vi "Breakdown Acoustics Controls.vi"() -> ()   [LabVIEW 2013]
doc: "Recommended Input Signal: 10 Hz, 1.8 Vpp, sine wave\n\nThis example requires NI-Scope 3.3 or later.\nDevices Supported: NI 5112, NI 5620, NI 5621, NI 5122, NI 5124, NI 5922, NI 5114, NI 5142\n\nVI Description:\n\nThis example demonstrates using continuous acquisition to fetch a user-defined, but quite large record of data all while continuously streaming the data to a binary file using the Win32 File I/O VIs. The digitizer is configured using the Configure Vertical and Configure Horizontal VI's. Auto setup in this case may not be useful, as it may choose a horizontal rate that exceeds the computer's streaming capabilities.\n\nIn this example, continuous acquisition is used. This allows the user to start the digitizer, and continuously fetch data without losing any points. This is accomplished by configuring a software trigger and never sending the software trigger. Therefore, the digitizer will continuously acquire data into its onboard memory until Abort or Close is called.\n\nThe producer loop continuously fetches data from onboard memory into the LabVIEW memory using DMA transfers. This data is placed into a queue in order to efficiently transfer the data to a parallel consumer loop where it is written file. If the sampling rate is low, the computer can fetch all the data from the digitizer, so data is never overwritten. However, at faster sampling rates, the computer will not be able to fetch the data before it is overwritten by new data. This results in the \"data overwritten\" error.\n\nThe consumer loop continuously empties data from the queue and writes data to disk using the Win32 Write File.vi. The file is opened using the Win32 Open File.vi, which disables Windows caching during the write process, resulting in increased performance. However when Windows caching is disabled, <b>data must be written to file in a multiple of the sector size of the disk (typically 512 bytes).</b>"
uses:
  <vilib>/Utility/error.llb/DialogType.ctl
  Breakdown Acoustics Controls/UDP Heartbeat Globals.vi
  <vilib>/Waveform/WDTFileIO.llb/ Write Waveforms to File (1D).vi
  Breakdown Acoustics Controls.lvlib
panel:
  out "Spark!":bool
  out "Spark Flag Updater\nHeartbeat":bool
  out "# DAQ Restarts":i32
  out "# Triggers":i32
  in  "Force Trigger":bool
  out "Triggered":bool
  in  "Tab Control":T1(tab)
  in  "Max Queue Size":i32=8
  in  "Samples Per Channel":i32=5120 caption="Max Points Per Fetch" step=1048576
  in  "Configuration File":path=path "\\\\beams-utility\\mta_archive$/mtarflv_shared/Microphone DAQ/LabVIEW/VI/Shared/SCM_without_Cu_windows_cfg.xml"
  in  "Sample Rate":i32=100000
  in  "Queue Timeout (ms)":i32=100
  out "Data Directory":path
  in  "Reset Avg. RF Hammer Graph":bool
  in  "Reset Raw Signals Graph":bool
  in  "Reset Processed Signals Graph":bool
  out "Processed Signals":waveform(dbl)[](graph)
  out "Avg. RF Hammer":waveform(dbl)[](graph)
  out "Raw Signals":waveform(dbl)[](graph)
  out "# Microphones":i32
  in  "stop":bool
  out "Acquisition Status":bool
  # "Configuration Settings"
  # "Acquisition Settings"
  # "(should be a multiple of disk sector size)"
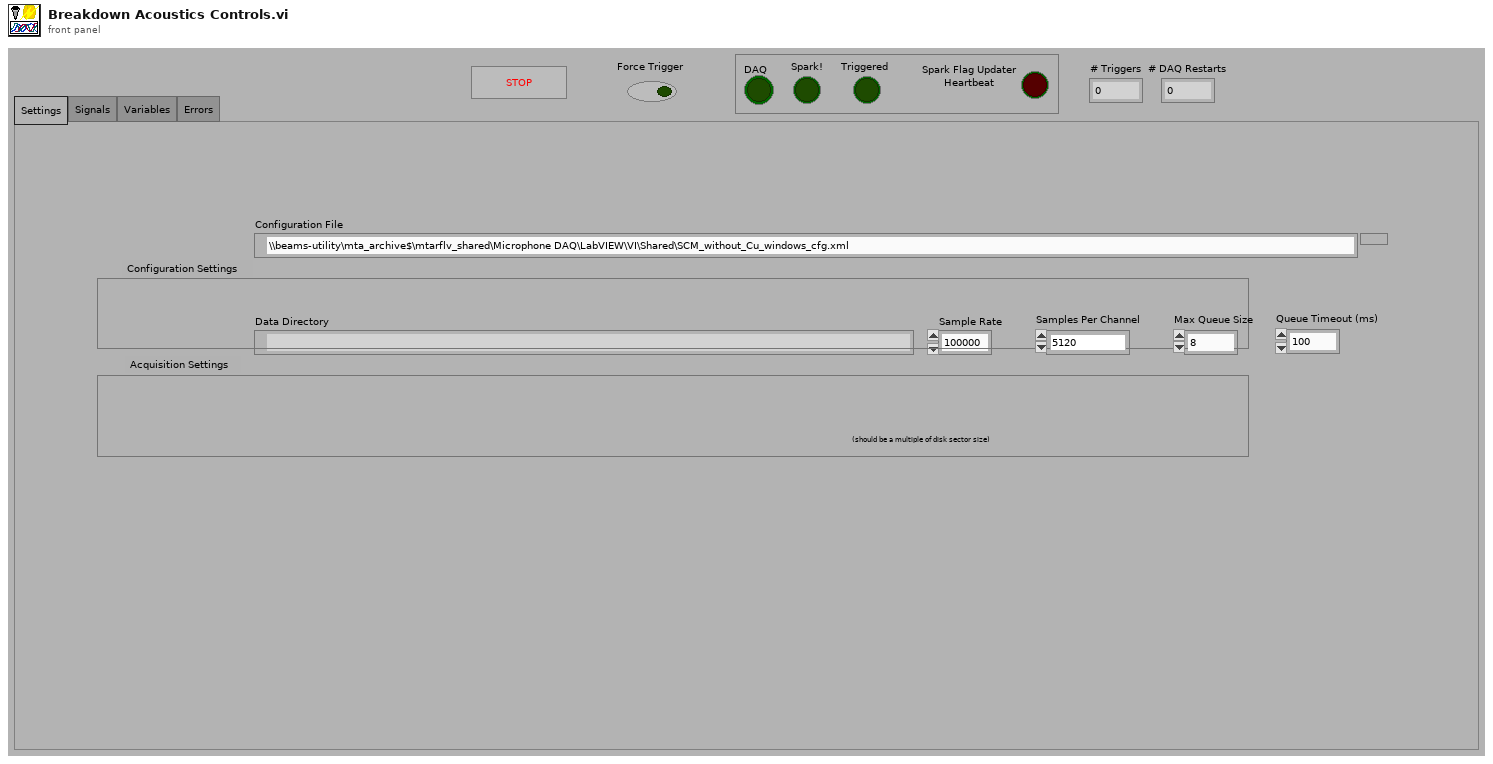
[diagram p1: front panel]
types:
  T1 = enum32{"Settings", "Signals", "Variables", "Errors"}
  T2 = typedef "DialogType.ctl" = u16
  T3 = cluster{"X Scale.Range:Minimum":dbl, "Y Scale.Range:Minimum":dbl, "X Scale.Range:Maximum":dbl, "Y Scale.Range:Maximum":dbl}
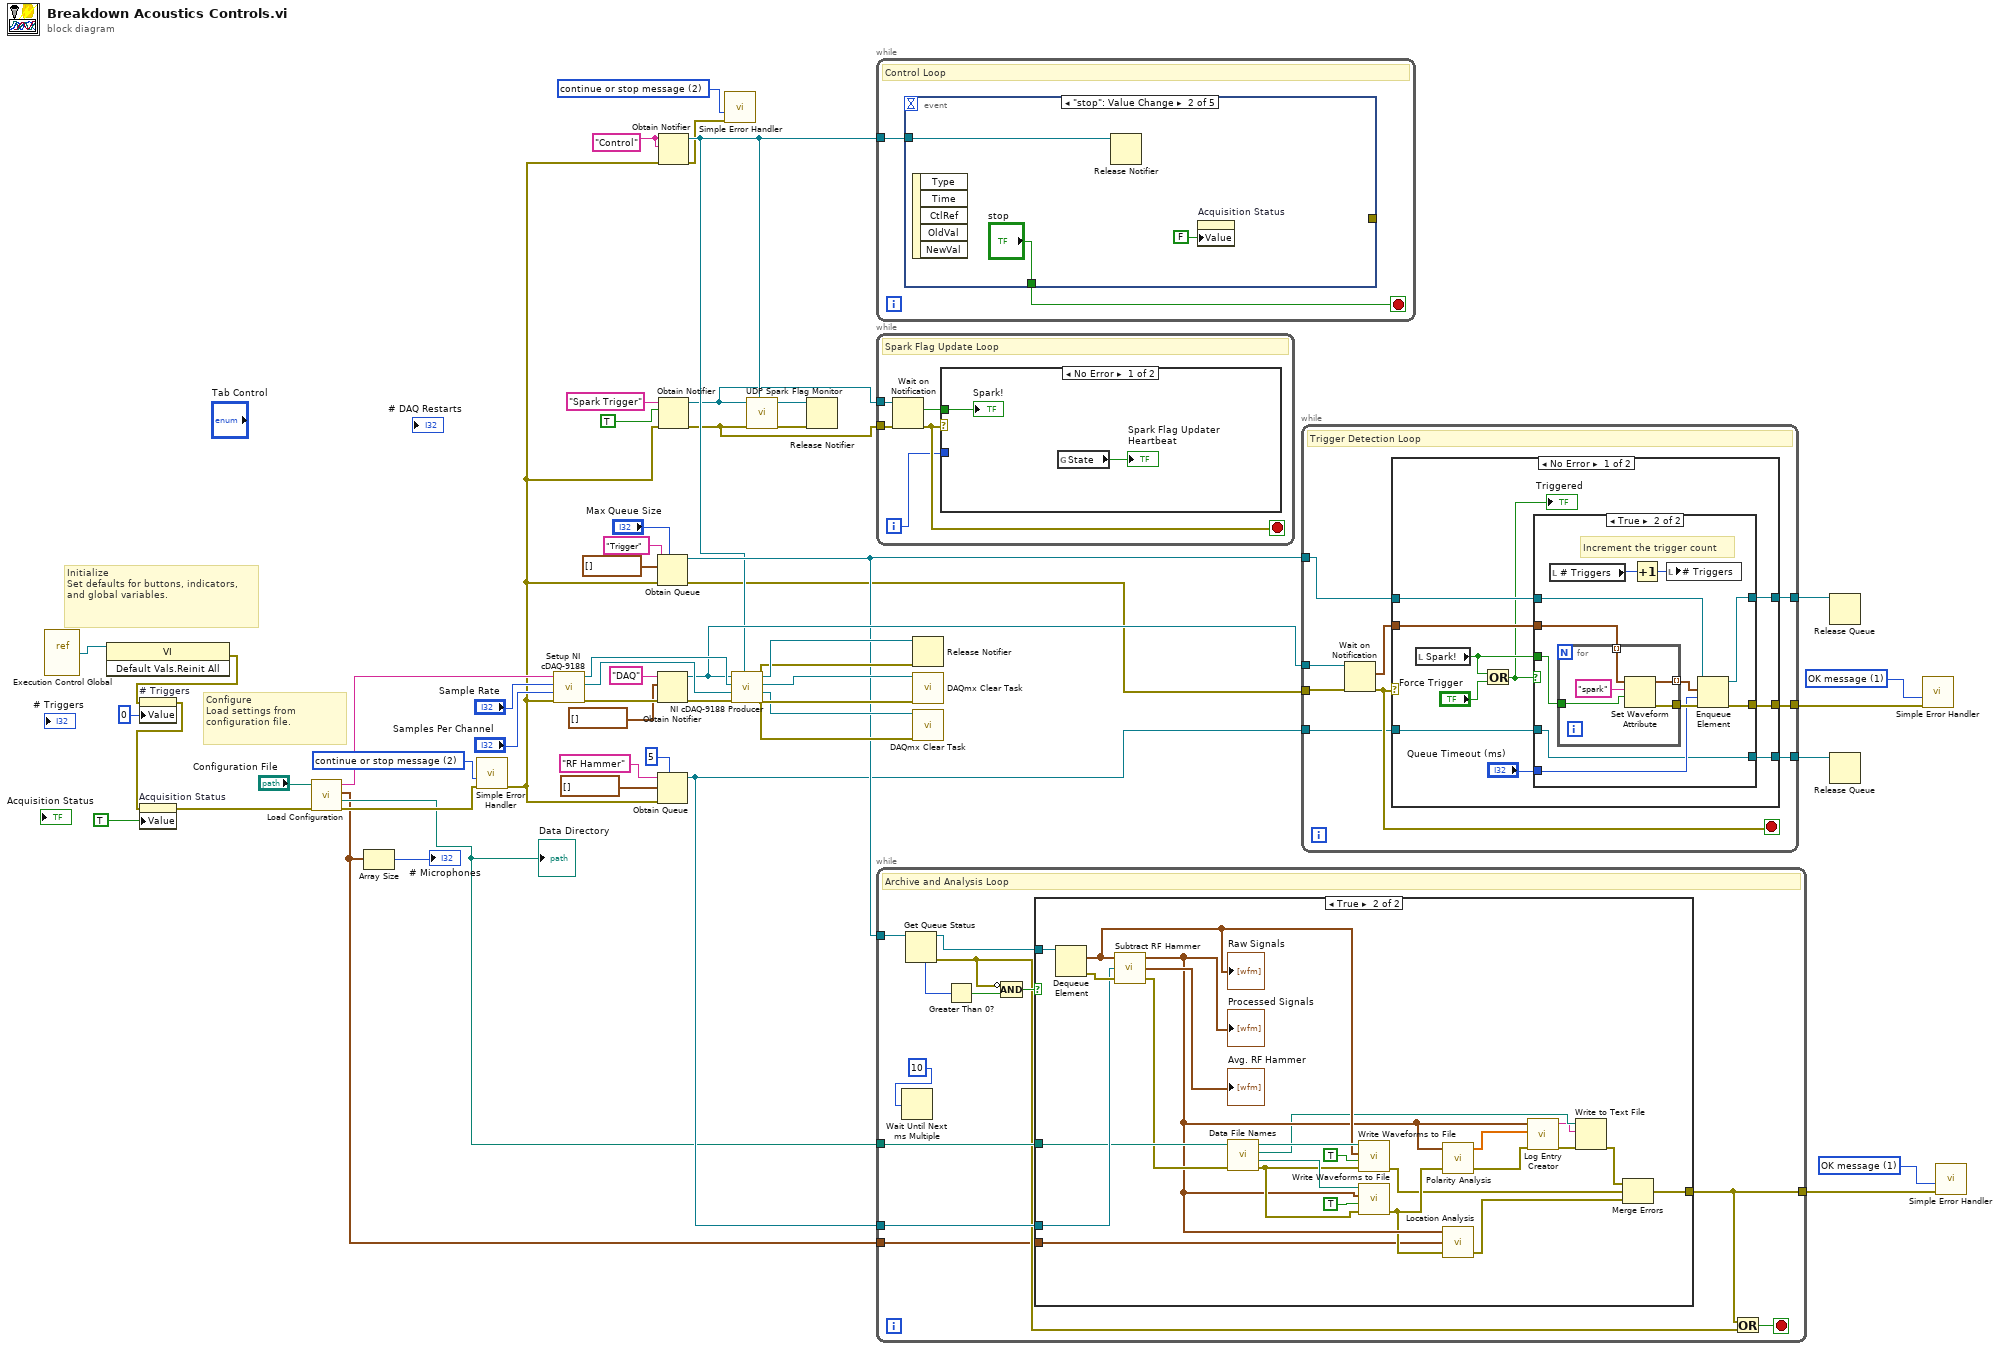
[diagram p0: block diagram]
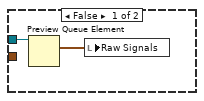
[diagram p2: hidden frame]
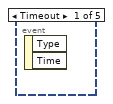
[diagram p3: hidden frame]
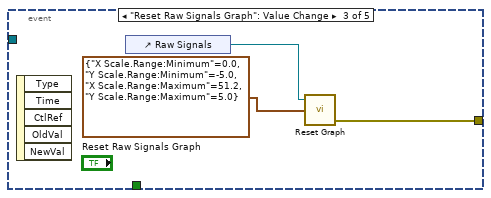
[diagram p4: hidden frame]
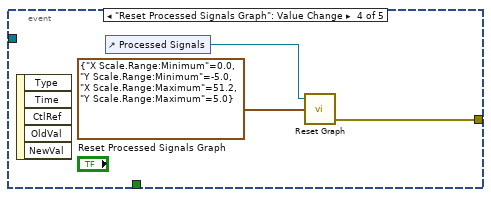
[diagram p5: hidden frame]
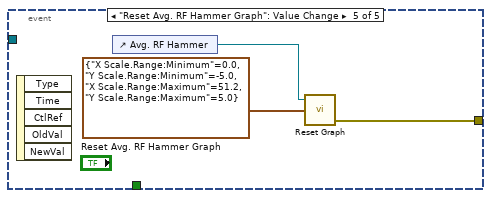
[diagram p6: hidden frame]
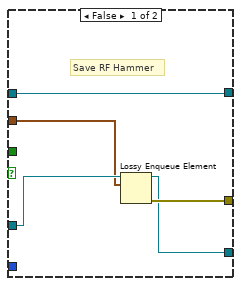
[diagram p8: hidden frame]
diagram:
  w1 = T2 1 items=["no dialog", "OK message", "continue or stop message", "OK message + warnings", "continue/stop + warnings"] ("type of dialog (OK msg:1)")
  w5 = T2 1 items=["no dialog", "OK message", "continue or stop message", "OK message + warnings", "continue/stop + warnings"] ("type of dialog (OK msg:1)")
  w10 = T2 2 items=["no dialog", "OK message", "continue or stop message", "OK message + warnings", "continue/stop + warnings"] ("type of dialog (OK msg:1)")
  w31 = "Control" ("name (unnamed)")
  w50 = T2 2 items=["no dialog", "OK message", "continue or stop message", "OK message + warnings", "continue/stop + warnings"] ("type of dialog (OK msg:1)")
  # "Configure\nLoad settings from configuration file."
  # "Initialize\nSet defaults for buttons, indicators, and global variables."
  n1 = vi-ref "Execution Control Global.vi"() -> (w44:refnum<vi>)
  n2 = invoke class="VI" method="Default Vals.Reinit All"(reference=w44) -> (error out=w43:errorcluster)  [unwired: 2 in, 2 out]
  n3 = property on="# Triggers" class="DigNum (strict)"(error in=w43, "Value"=0 ("# Triggers")) -> (error out=w19:errorcluster)  [unwired: 1 in, 1 out]
  n4 = property on="Acquisition Status" class="Bool (strict)"(error in=w19, "Value"=TRUE ("Acquisition Status")) -> (error out=w45:errorcluster)  [unwired: 1 in, 1 out]
  n5 = call "Load Configuration.vi"("error in"=w45, "Configuration File"="Configuration File") -> ("error out"=w30:errorcluster, "Data Directory"=w4:path, "Microphone Locations"=w3:cluster{"r":dbl, "theta":dbl, "z":dbl}[], "DAQ Channels"=w40:string)  [unwired: 6 in]
  "Data Directory" <- w4
  n6 = Array Size(array=w3) -> (size(s)=→"# Microphones":i32)
  n7 = call <vilib>:"Simple Error Handler.vi"("type of dialog (OK msg:1)"=w50, "error in (no error)"=w30) -> ("error out"=w24:errorcluster)  [unwired: 3 in, 4 out]
  n8 = call "Setup NI cDAQ-9188.vi"("error in"=w24, "Samples per Channel"="Samples Per Channel", "Sample Rate"="Sample Rate", "Physical Channels"=w40) -> ("error out"=w37:errorcluster, "Counter Task"=w34:refnum<k21>, "AI Voltage Task"=w33:refnum<k21>)  [unwired: 5 in]
  n9 = Obtain Queue(max queue size (-1, unlimited)="Max Queue Size", name (unnamed)="Trigger", element data type=waveform(dbl)[] [], error in (no error)=w24) -> (queue out=w18:refnum<queue>, error out=w11:errorcluster)  [unwired: 1 in, 1 out]
  n10 = Obtain Notifier(name (unnamed)="DAQ", notification data type=waveform(dbl)[] [] ("data"), error in (no error)=w37) -> (notifier out=w27:refnum<notifier>, error out=w35:errorcluster)  [unwired: 1 in, 1 out]
  n11 = Obtain Queue(max queue size (-1, unlimited)=5, name (unnamed)="RF Hammer", element data type=waveform(dbl)[] [], error in (no error)=w24) -> (queue out=w17:refnum<queue>)  [unwired: 1 in, 2 out]
  n12 = Obtain Notifier(name (unnamed)=w31, notification data type=w31, error in (no error)=w24) -> (notifier out=w16:refnum<notifier>, error out=w9:errorcluster)  [unwired: 1 in, 1 out]
  n13 = Obtain Notifier(name (unnamed)="Spark Trigger", notification data type=TRUE, error in (no error)=w24) -> (notifier out=w15:refnum<notifier>, error out=w12:errorcluster)  [unwired: 1 in, 1 out]
  n14 = call <vilib>:"Simple Error Handler.vi"("type of dialog (OK msg:1)"=w10, "error in (no error)"=w9) -> ()  [unwired: 3 in, 5 out]
  n15 = call "NI cDAQ-9188 Producer.vi"("Control Notifier"=w16, "error in"=w35, "Counter Task"=w34, "AI Voltage Task"=w33, "DAQ Notifier"=w27) -> ("error out"=w21:errorcluster, "Counter Task out"=w20:refnum<k21>, "AI Voltage Task out"=w22:refnum<k21>, "DAQ Notifier out"=w23:refnum<notifier>)  [unwired: 3 in]
  n16 = call "UDP Spark Flag Monitor.vi"("Control Notifier"=w16, "error in (no error)"=w12, "Spark Status Notifier"=w15) -> ("error out"=w13:errorcluster, "Spark Status Notifier out"=w14:refnum<notifier>)  [unwired: 7 in]
  n17 = Release Notifier(notifier=w14, error in (no error)=w13) -> ()  [unwired: 1 in, 3 out]
  n18 = while {
    tunnel: w16 -> [w53]
    stop <- w54 stop-if-true
    # "Control Loop"
    n19 = event shown="[1] \"stop\": Value Change" {
      selector: _ -> [_ _ _ _ _]
      dyn-events: _ -> [_ _ _ _ _]
      timeout: _ -> [_ _ _ _ _]
      tunnel: [_ _ w58 w61 w64] -> _
      tunnel: [_ "stop" _ _ _] -> w54
      tunnel: w53 -> [_ w56 _ _ _]
      event Timeout {
        n20 = event-data() -> ()  [unwired: 1 in, 2 out]
      }
      event "stop": Value Change {
        n21 = event-data() -> ()  [unwired: 1 in, 5 out]
        n22 = Release Notifier(notifier=w56) -> ()  [unwired: 2 in, 3 out]
        n23 = property on="Acquisition Status" class="Bool (strict)"("Value"=FALSE ("Acquisition Status")) -> ()  [unwired: 2 in, 2 out]
      }
      event "Reset Raw Signals Graph": Value Change {
        n24 = event-data() -> ()  [unwired: 1 in, 5 out]
        n25 = control-ref of="Raw Signals"() -> (w60:refnum<vi>)
        n26 = call "Reset Graph.vi"("Graph Boundaries"=T3 {"X Scale.Range:Minimum"=0.0, "Y Scale.Range:Minimum"=-5.0, "X Scale.Range:Maximum"=51.2, "Y Scale.Range:Maximum"=5.0}, "Graph Reference"=w60) -> ("error out"=w58:errorcluster)  [unwired: 3 in]
      }
      event "Reset Processed Signals Graph": Value Change {
        n27 = event-data() -> ()  [unwired: 1 in, 5 out]
        n28 = control-ref of="Processed Signals"() -> (w62:refnum<vi>)
        n29 = call "Reset Graph.vi"("Graph Boundaries"=T3 {"X Scale.Range:Minimum"=0.0, "Y Scale.Range:Minimum"=-5.0, "X Scale.Range:Maximum"=51.2, "Y Scale.Range:Maximum"=5.0}, "Graph Reference"=w62) -> ("error out"=w61:errorcluster)  [unwired: 3 in]
      }
      event "Reset Avg. RF Hammer Graph": Value Change {
        n30 = event-data() -> ()  [unwired: 1 in, 5 out]
        n31 = control-ref of="Avg. RF Hammer"() -> (w66:refnum<vi>)
        n32 = call "Reset Graph.vi"("Graph Boundaries"=T3 {"X Scale.Range:Minimum"=0.0, "Y Scale.Range:Minimum"=-5.0, "X Scale.Range:Maximum"=51.2, "Y Scale.Range:Maximum"=5.0}, "Graph Reference"=w66) -> ("error out"=w64:errorcluster)  [unwired: 3 in]
      }
    }
  }
  n33 = while {
    tunnel: w15 -> [w71]
    tunnel: w12 -> [w69]
    i -> [w67]
    stop <- w70 stop-if-true
    # "Spark Flag Update Loop"
    n34 = Wait on Notification(notifier=w71, error in (no error)=w69) -> (notification=w68:bool, error out=w70:errorcluster)  [unwired: 4 out]
    n35 = case shown="No Error" w70 {
      tunnel: w68 -> [w73 _]
      tunnel: w67 -> [_ _]
      frame No Error {
        n36 = global read "UDP Heartbeat Globals.vi" "State"() -> (→"Spark Flag Updater\nHeartbeat":bool)
        "Spark!" <- w73
      }
      frame Error {
      }
    }
  }
  n37 = while {
    tunnel: w18 -> [w85]
    tunnel: w17 -> [w81]
    tunnel: w4 -> [w80]
    tunnel: w3 -> [w75]
    tunnel: [w74] -> w2
    stop <- w77 stop-if-true
    # "Archive and Analysis Loop"
    n38 = Wait Until Next ms Multiple(millisecond multiple=u32 10) -> ()  [unwired: 1 out]
    n39 = Get Queue Status(queue=w85) -> (queue out=w83:refnum<queue>, error out=w76:errorcluster, # elements in queue=w84:i32)  [unwired: 2 in, 5 out]
    n40 = Greater Than 0?(x=w84) -> (x > 0?=w79:bool)
    n41 = Compound Arithmetic op=AND(invert w76, w79) -> (w78:bool)
    n42 = case shown="True" w78 {
      tunnel: w83 -> [_ w111]
      tunnel: w81 -> [w87 w109]
      tunnel: w80 -> [_ w106]
      tunnel: [_ w93] -> w74
      tunnel: w75 -> [_ w88]
      frame False {
        n43 = Preview Queue Element(queue=w87) -> (element=w86:waveform(dbl)[])  [unwired: 2 in, 3 out]
        n44 = local write "Raw Signals"(w86) -> ()
      }
      frame True {
        n45 = Dequeue Element(queue=w111) -> (element=w100:waveform(dbl)[], error out=w110:errorcluster)  [unwired: 2 in, 2 out]
        "Raw Signals" <- w100
        n46 = call "Subtract RF Hammer.vi"("error in (no error)"=w110, "RF Hammer Queue"=w109, "Breakdown Signal"=w100) -> ("error out"=w105:errorcluster, "Average RF Hammer"=→"Avg. RF Hammer":waveform(dbl)[], "Reduced Signal"=w97:waveform(dbl)[])
        "Processed Signals" <- w97
        n47 = call "Data File Names.vi"("error in (no error)"=w105, "Data Directory"=w106) -> ("error out"=w101:errorcluster, "Reduced Data File"=w102:path, "Log File"=w92:path, "Raw Data File"=w104:path)  [unwired: 6 in]
        n48 = call-poly <vilib>:"Write Waveforms to File.vi"("error in (no error)"=w101, "append to file? (new file:F)"=TRUE, "waveform array"=w100, "file path (dialog if empty)"=w104) -> ("error out"=w95:errorcluster)  [unwired: 6 in, 1 out]
        n49 = call-poly <vilib>:"Write Waveforms to File.vi"("error in (no error)"=w101, "append to file? (new file:F)"=TRUE, "waveform array"=w97, "file path (dialog if empty)"=w102) -> ("error out"=w96:errorcluster)  [unwired: 6 in, 1 out]
        n50 = call "Polarity Analysis.vi"("error in (no error)"=w96, "Raw Signals"=w97) -> ("error out"=w98:errorcluster, "Signal Integrations"=w99:dbl[])  [unwired: 2 in]
        n51 = call "Location Analysis.vi"("error in (no error)"=w96, "Microphone Locations"=w88, "Signals"=w97) -> ("error out"=w94:errorcluster)  [unwired: 2 in]
        n52 = call "Log Entry Creator.vi"("error in (no error)"=w98, "Signal Integration Values"=w99, "Waveforms"=w97) -> ("error out"=w90:errorcluster, "Log Entry"=w91:string)  [unwired: 7 in]
        n53 = Write to Text File(file (use dialog)=w92, text=w91, error in=w90) -> (error out=w89:errorcluster)  [unwired: 1 in, 2 out]
        n54 = Merge Errors(w89, w95, w94) -> (w93:errorcluster)
      }
    }
    n55 = Or(x=w74, y=w76) -> (x .or. y?=w77:bool)
  }
  n56 = Release Notifier(notifier=w23, error in (no error)=w21) -> ()  [unwired: 1 in, 3 out]
  n57 = call <vilib>:"DAQmx Clear Task.vi"("task in"=w22, "error in"=w21) -> ()  [unwired: 13 in, 1 out]
  n58 = call <vilib>:"DAQmx Clear Task.vi"("task in"=w20, "error in"=w21) -> ()  [unwired: 13 in, 1 out]
  n59 = while {
    tunnel: w27 -> [w120]
    tunnel: w11 -> [w118]
    tunnel: w18 -> [w117]
    tunnel: w17 -> [w115]
    tunnel: [w114] -> w6
    tunnel: [w113] -> w8
    tunnel: [w112] -> w7
    stop <- w119 stop-if-true
    # "Trigger Detection Loop"
    n60 = Wait on Notification(notifier=w120, error in (no error)=w118) -> (notification=w116:waveform(dbl)[], error out=w119:errorcluster)  [unwired: 4 out]
    n61 = case shown="No Error" w119 {
      selector: w119 -> [_ w152]
      tunnel: w117 -> [w129 w154]
      tunnel: w116 -> [w130 _]
      tunnel: w115 -> [w127 w153]
      tunnel: [w126 w152] -> w114
      tunnel: [w125 w154] -> w113
      tunnel: [w124 w153] -> w112
      frame No Error {
        n62 = local read "Spark!"() -> (w122:bool)
        n63 = Or(x=w122, y="Force Trigger") -> (x .or. y?=w121:bool)
        "Triggered" <- w121
        n64 = case shown="True" w121 {
          tunnel: w130 -> [w134 w146]
          tunnel: w129 -> [w133 w145]
          tunnel: "Queue Timeout (ms)" -> [_ w142]
          tunnel: w127 -> [w135 w139]
          tunnel: [w132 w141] -> w126
          tunnel: [w133 w140] -> w125
          tunnel: [w131 w139] -> w124
          tunnel: w122 -> [_ w138]
          frame False {
            # "Save RF Hammer"
            n65 = Lossy Enqueue Element(queue=w135, element=w134) -> (queue out=w131:refnum<queue>, error out=w132:errorcluster)  [unwired: 1 in, 2 out]
          }
          frame True {
            # "Increment the trigger count"
            n66 = local read "# Triggers"() -> (w136:i32)
            n67 = for {
              tunnel: w146 -> [w150] mode=indexing
              tunnel: [w149] -> w144 mode=indexing
              tunnel: [w148] -> w143
              tunnel: w138 -> [w147]
              n68 = Set Waveform Attribute(5:w147, 6:"spark" ("name"), 7:w150) -> (0:w148:errorcluster, 3:w149:waveform(dbl))  [unwired: 1 in, 1 out]
            }
            n69 = Increment(x=w136) -> (x+1=w137:i32)
            n70 = local write "# Triggers"(w137) -> ()
            n71 = Enqueue Element(queue=w145, element=w144, timeout in ms (-1)=w142, error in (no error)=w143) -> (queue out=w140:refnum<queue>, error out=w141:errorcluster)  [unwired: 1 out]
          }
        }
      }
      frame Error {
      }
    }
  }
  n72 = Release Queue(queue=w8) -> ()  [unwired: 2 in, 3 out]
  n73 = Release Queue(queue=w7) -> ()  [unwired: 2 in, 3 out]
  n74 = call <vilib>:"Simple Error Handler.vi"("type of dialog (OK msg:1)"=w5, "error in (no error)"=w6) -> ()  [unwired: 3 in, 5 out]
  n75 = call <vilib>:"Simple Error Handler.vi"("type of dialog (OK msg:1)"=w1, "error in (no error)"=w2) -> ()  [unwired: 3 in, 5 out]
